vi "FF_Platform.vi"(8 "error in (no error)":errorcluster, 9 "WristVelocity":dbl[](array[numeric]), 10 "WristPosition":dbl[](array[numeric]), 11 "Force Field Controller in":refnum<class "ForceField.lvclass">) -> (0 "error out":errorcluster, 1 "ClosestPt":dbl[](array[numeric]), 2 "Force":dbl[](array[numeric]), 3 "Force Field Controller out":refnum<class "ForceField.lvclass">, 4 "ForceComp":dbl[](array[numeric]))   [LabVIEW 2015, in "ForceField.lvclass"]
uses:
  ForceField.lvclass
  ForceField.lvclass/ForceField.ctl
  TypeDef/TND.ctl
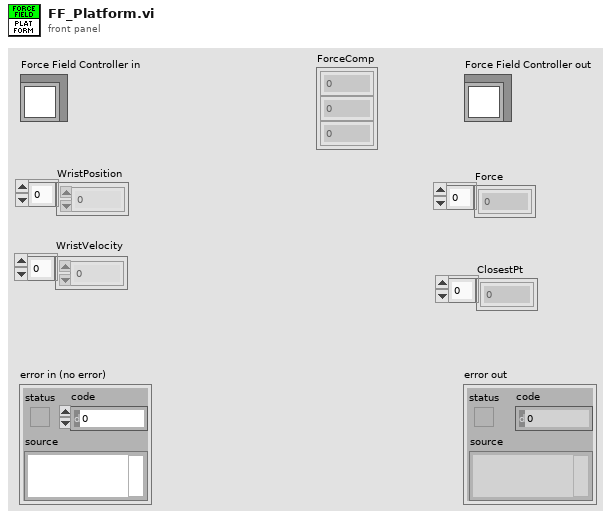
[diagram p1: front panel]
types:
  T1 = typedef "ForceField.lvclass/TND.ctl" = cluster{"Vt":dbl[], "Vn":dbl[], "Dmin":dbl}
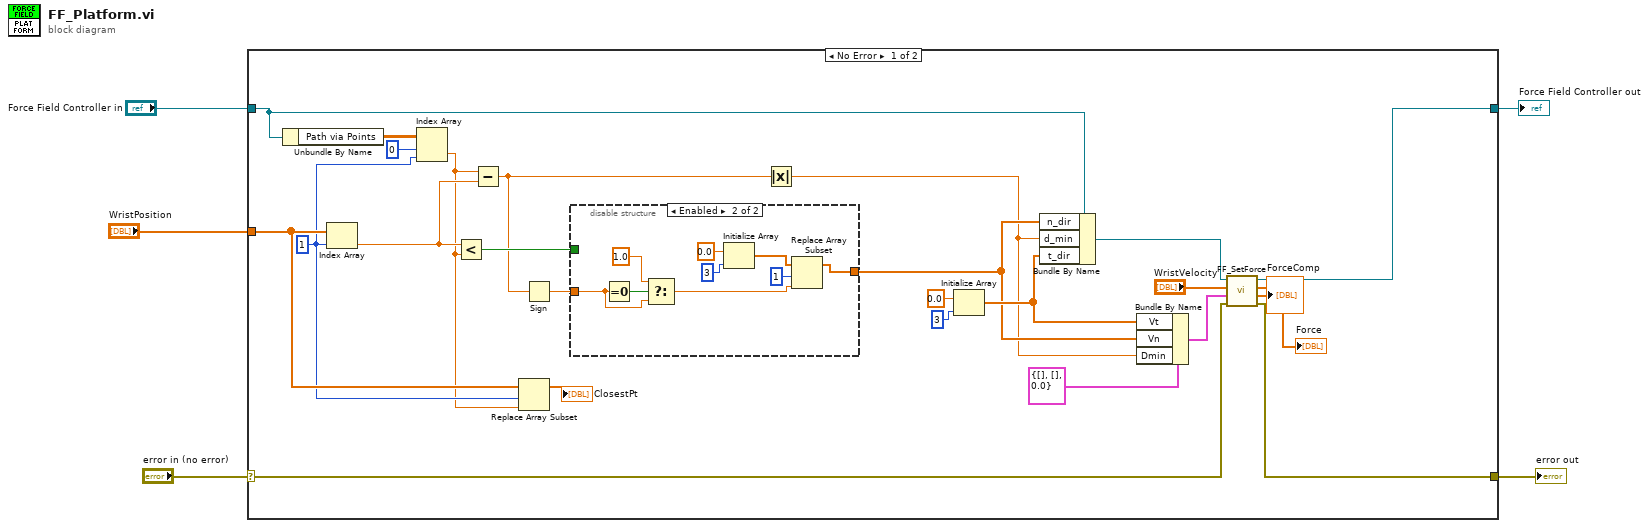
[diagram p0: block diagram]
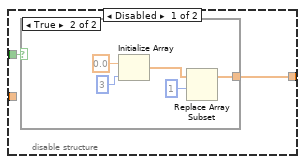
[diagram p2: hidden frame]
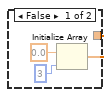
[diagram p3: hidden frame]
diagram:
  n1 = case shown="No Error" "error in (no error)" {
    selector: "error in (no error)" -> [w20 w51]
    tunnel: [w19 w51] -> w4
    tunnel: [w22 w50] -> w2
    tunnel: "Force Field Controller in" -> [w28 w50]
    tunnel: "WristPosition" -> [w15 _]
    frame No Error {
      w14 = 1 ("disabled index (col)")
      n2 = Unbundle By Name(w28) -> ("Path via Points"=w30:dbl[][])
      n3 = Index Array(array=w15, index=w14) -> (element=w26:dbl)
      n4 = Index Array(array=w30, index (row)=0, index (col)=w14) -> (element=w13:dbl)
      n5 = Less?(x=w26, y=w13) -> (x < y?=w27:bool)
      n6 = Subtract(x=w13, y=w26) -> (x-y=w17:dbl)
      n7 = Replace Array Subset(array=w15, new element=w13, index=w14) -> (→"ClosestPt":dbl[])
      n8 = Sign(1:w17) -> (0:w16:dbl)
      n9 = disable-structure shown="Enabled" {
        disable-tunnel: w27 -> [w32 _]
        disable-tunnel: [w31 w45] -> w8
        disable-tunnel: w16 -> [_ w42]
        frame Disabled {
          n10 = case shown="True" w32 {
            tunnel: [w34 w36] -> w31
            frame False {
              n11 = Initialize Array(0.0 ("element"), 3 ("dimension size")) -> (w34:dbl[])
            }
            frame True {
              n12 = Initialize Array(0.0 ("element"), 3 ("dimension size")) -> (w38:dbl[])
              n13 = Replace Array Subset(array=w38, index=1) -> (w36:dbl[])  [unwired: 1 in]
            }
          }
        }
        frame Enabled {
          n14 = Equal To 0?(x=w42) -> (x = 0?=w44:bool)
          n15 = Select(t=1.0, s=w44, f=w42) -> (s? t:f=w43:dbl)
          n16 = Initialize Array(0.0 ("element"), 3 ("dimension size")) -> (w47:dbl[])
          n17 = Replace Array Subset(array=w47, new element=w43, index=1) -> (w45:dbl[])
        }
      }
      n18 = Absolute Value(x=w17) -> (abs(x)=w7:dbl)
      n19 = Initialize Array(0.0 ("element"), 3 ("dimension size")) -> (w9:dbl[])
      n20 = Bundle By Name(cluster=w28, "n_dir"=w8, "d_min"=w7, "t_dir"=w9) -> (w23:refnum<class "ForceField.lvclass">)
      n21 = Bundle By Name(cluster=T1 {"Vt"=[], "Vn"=[], "Dmin"=0.0} ("TND"), "Vt"=w9, "Vn"=w8, "Dmin"=w7) -> (w6:T1)
      n22 = call "FF_SetForce.vi"("error in (no error)"=w20, "TND"=w6, "AnkleVelocity"="WristVelocity", "Force Field Controller in"=w23) -> ("error out"=w19:errorcluster, "ForceNTD"=→"ForceComp":dbl[], "ForceXYZ"=→"Force":dbl[], "Force Field Controller out"=w22:refnum<class "ForceField.lvclass">)  [unwired: 4 in]
    }
    frame Error {
    }
  }
  "error out" <- w4
  "Force Field Controller out" <- w2
